vi "IsTeamNearBall.vi"(0 "Events in":refnum<class "Events.lvclass">, 5 "TeamRobots":refnum<class "Robot.lvclass">[](array[class]), 7 "Ball":refnum<class "Ball.lvclass">, 9 "DistanceToBallPos":dbl, 11 "error in (no error)":errorcluster) -> (4 "Events out":refnum<class "Events.lvclass">, 6 "possession":bool, 8 "idPossession":i32, 15 "error out":errorcluster)   [LabVIEW 2023, in "Events.lvclass"]
uses:
  Events.lvclass
  Robot_class/Robot.lvclass
  Ball_class/Ball.lvclass
  Robot_class/Robot.lvclass/Robot.ctl
  Robot_class/Read id.vi
  Utilities_class/Utilities.lvclass
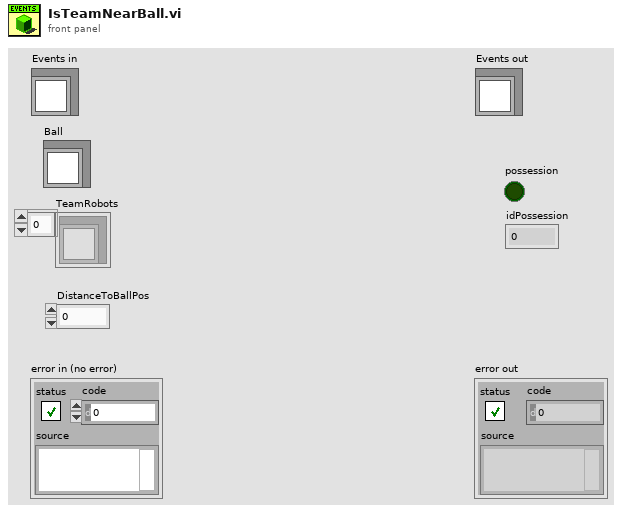
[diagram p1: front panel]
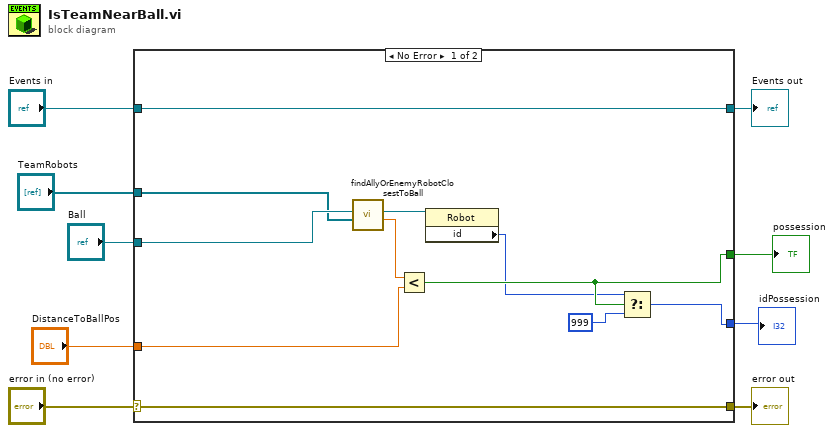
[diagram p0: block diagram]
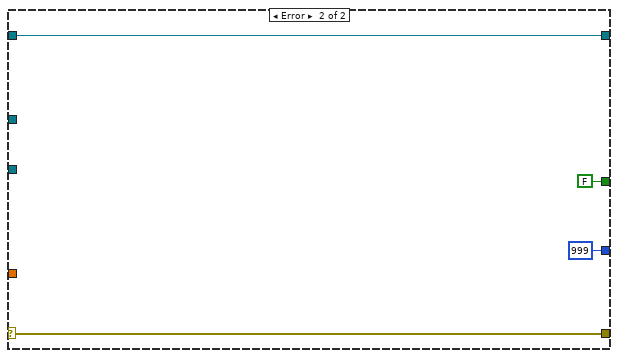
[diagram p2: hidden frame]
diagram:
  n1 = case shown="No Error" "error in (no error)" {
    selector: "error in (no error)" -> [w19 w24]
    tunnel: [w19 w24] -> w8
    tunnel: [w20 w23] -> w6
    tunnel: "Events in" -> [w20 w23]
    tunnel: "TeamRobots" -> [w17 _]
    tunnel: "Ball" -> [w18 _]
    tunnel: [w13 FALSE] -> w3
    tunnel: [w11 999] -> w2
    tunnel: "DistanceToBallPos" -> [w14 _]
    frame No Error {
      n2 = call "findAllyOrEnemyRobotClosestToBall.vi"("Ally/Enemy Robots"=w17, "Ball"=w18) -> ("Robot distance to ball"=w15:dbl, "Robot"=w16:refnum<class "Robot.lvclass">)  [unwired: 6 in, 2 out]
      n3 = Less?(x=w15, y=w14) -> (x < y?=w13:bool)
      n4 = property class="Robot"(reference=w16) -> ("id"=w12:i32)  [unwired: 1 in, 2 out]
      n5 = Select(t=w12, s=w13, f=999) -> (s? t:f=w11:i32)
    }
    frame Error {
    }
  }
  "error out" <- w8
  "Events out" <- w6
  "possession" <- w3
  "idPossession" <- w2
